vi "Write Error Status (Array).vi"(8 "error in":errorcluster, 10 "Errors":errorcluster[](array[cluster]), 11 "Cycler in":refnum<class "Cycler.lvclass">) -> (0 "error out":errorcluster, 3 "Cycler out":refnum<class "Cycler.lvclass">)   [LabVIEW 2023, in "Cycler.lvclass"]
uses:
  Cycler.lvclass
  Cycler.lvclass/Cycler.ctl
  <vilib>/ADAS Replay HIL/Channels/Tag Wrapper/Polymorphic/Write Channel (I32).vi
  <vilib>/ADAS Replay HIL/Channels/Tag Wrapper/Polymorphic/Write Channel (I32).vi/cccb8e89-591f-4bb4-9d4e-ae06ba1f5498.vi
  <vilib>/ADAS Replay HIL/Channels/Tag Wrapper/Polymorphic/Write Channel (I32).vi/cccb8e89-591f-4bb4-9d4e-ae06ba1f5498.vi/4bc1c15b-36ab-481f-b8dd-c64075ce723a.vi
  <vilib>/ADAS Replay HIL/Channels/Tag Wrapper/Polymorphic/Write Channel (I32).vi/cccb8e89-591f-4bb4-9d4e-ae06ba1f5498.vi/d83cb72b-7713-41fc-a3d1-682de79cf574.vi
  <vilib>/ADAS Replay HIL/Channels/Tag Wrapper/Tag Wrapper.lvlib
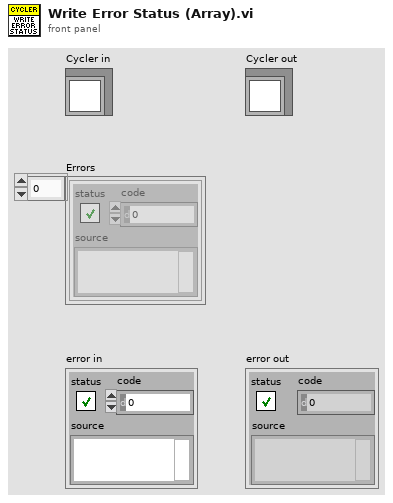
[diagram p1: front panel]
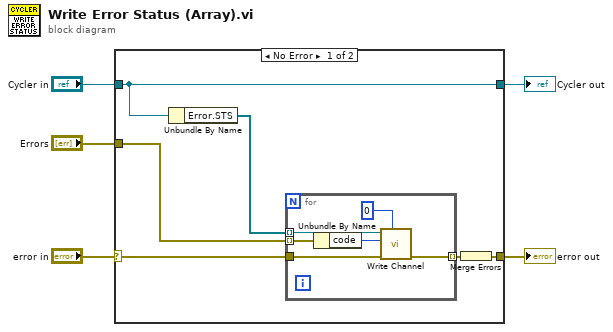
[diagram p0: block diagram]
diagram:
  n1 = case shown="No Error" "error in" {
    selector: "error in" -> [w9 w18]
    tunnel: [w6 w18] -> w4
    tunnel: [w11 w19] -> w2
    tunnel: "Cycler in" -> [w11 w19]
    tunnel: "Errors" -> [w7 _]
    frame No Error {
      n2 = Unbundle By Name(w11) -> ("Error.STS"=w8:refnum<k21>[])
      n3 = for {
        tunnel: w8 -> [w15] mode=indexing
        tunnel: w7 -> [w14] mode=indexing
        tunnel: w9 -> [w16]
        tunnel: [w17] -> w10 mode=indexing
        n4 = Unbundle By Name(w14) -> ("code"=w13:i32)
        n5 = call-poly <vilib>:"Write Channel.vi"("Timeout (ms)"=0, "error in"=w16, "Value to Write"=w13, "ADAS HIL Channel in"=w15) -> ("error out"=w17:errorcluster)  [unwired: 5 in, 2 out]
      }
      n6 = Merge Errors(w10) -> (w6:errorcluster)
    }
    frame Error {
    }
  }
  "error out" <- w4
  "Cycler out" <- w2
